vi "Angles to Robot.vi"(8 "Error In":errorcluster, 9 "Joint 2":dbl(slide)=83.34328358208955 scale=0.0..180.0, 10 "Joint 1":dbl(slide)=70.2089552238806 scale=0.0..180.0, 11 "Joint 0":dbl(slide)=0.44776119402984627 scale=0.0..180.0) -> (0 "Error Out":errorcluster, 3 "Angle array radians":dbl[](array[numeric]))   [LabVIEW 2015]
doc: "This VI converts all the angles of the simualtion to be at the same position as the servos of the robot."
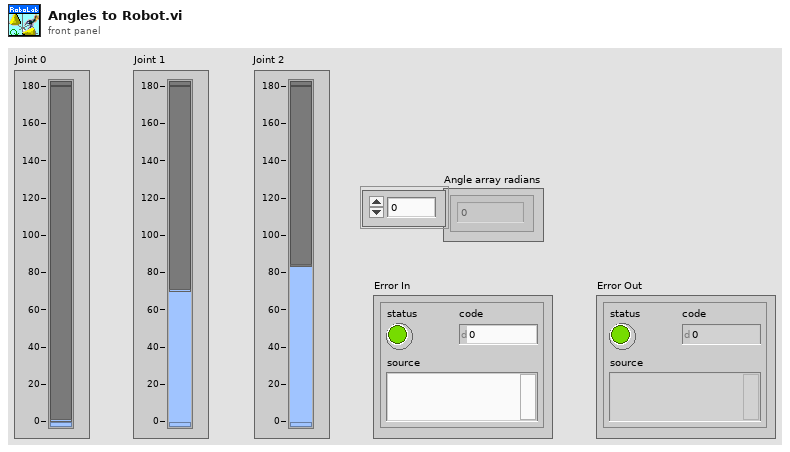
[diagram p1: front panel]
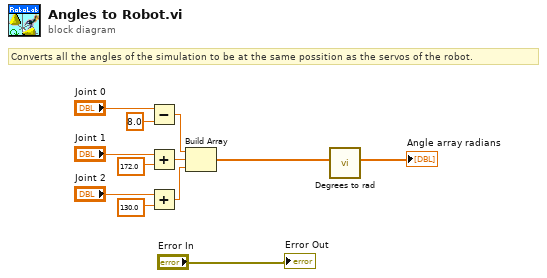
[diagram p0: block diagram]
diagram:
  # "Converts all the angles of the simulation to be at the same possition as the servos of the robot."
  n1 = Subtract(x="Joint 0", y=8.0) -> (x-y=w4:dbl)
  n2 = Add(x="Joint 1", y=172.0) -> (x+y=w5:dbl)
  n3 = Add(x="Joint 2", y=130.0) -> (x+y=w7:dbl)
  n4 = Build Array(w4, w5, w7) -> (w2:dbl[])
  n5 = call "Degrees to rad.vi"("Angle array Degrees"=w2) -> ("Angle array Radians"=→"Angle array radians":dbl[])  [unwired: 10 in]
  "Error Out" <- "Error In"
